vi "EPhysWork-Huet Model.vi"(3 "output control":T1, 4 "data":variant, 5 "X":dbl[](array[numeric]), 6 "a":dbl[](array[numeric])) -> (0 "error out":errorcluster, 1 "f'(X,a)":dbl[][](array[numeric]), 2 "f(X,a)":dbl[](array[numeric]))   [LabVIEW 2015]
doc: "Sum of three Gaussians, plus DC offset."
uses:
  <vilib>/gmath/NumericalOptimization/LM_output select.ctl
  <vilib>/gmath/NI_Gmath.lvlib
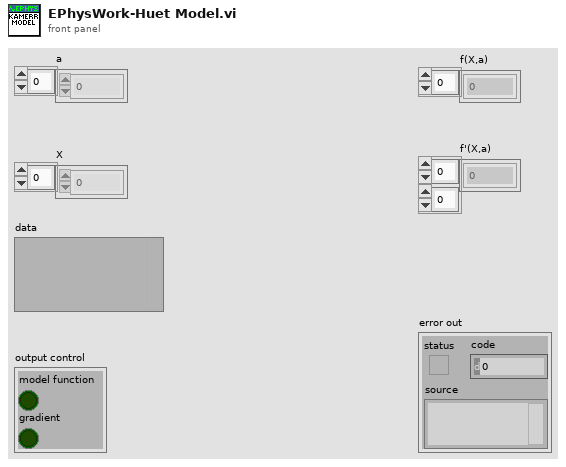
[diagram p1: front panel]
types:
  T1 = typedef "NI_Gmath.lvlib/LM_output select.ctl" = cluster{"model function":bool, "gradient":bool}
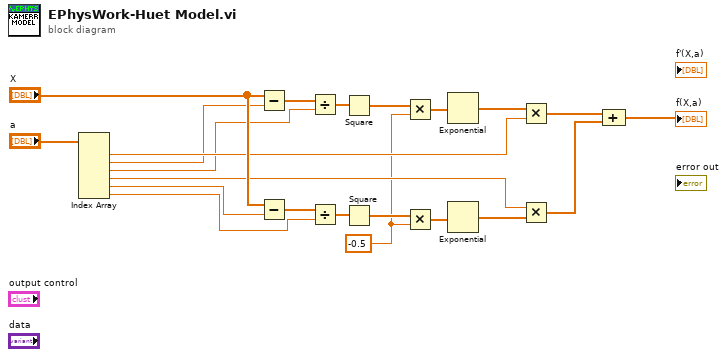
[diagram p0: block diagram]
diagram:
  w1 = -0.5
  n1 = Index Array(array="a") -> (element #1=w21:dbl, element #2=w20:dbl, element #3=w19:dbl, element #4=w18:dbl, element #5=w17:dbl, element #6=w16:dbl)  [unwired: 6 in]
  n2 = Subtract(x="X", y=w20) -> (x-y=w5:dbl[])
  n3 = Subtract(x="X", y=w17) -> (x-y=w4:dbl[])
  n4 = Divide(x=w5, y=w19) -> (x/y=w13:dbl[])
  n5 = Divide(x=w4, y=w16) -> (x/y=w10:dbl[])
  n6 = Square(x=w13) -> (x^2=w3:dbl[])
  n7 = Square(x=w10) -> (x^2=w2:dbl[])
  n8 = Multiply(x=w3, y=w1) -> (x*y=w7:dbl[])
  n9 = Multiply(x=w2, y=w1) -> (x*y=w6:dbl[])
  n10 = Exponential(1:w7) -> (0:w12:dbl[])
  n11 = Exponential(1:w6) -> (0:w11:dbl[])
  n12 = Multiply(x=w12, y=w21) -> (x*y=w9:dbl[])
  n13 = Multiply(x=w18, y=w11) -> (x*y=w8:dbl[])
  n14 = Compound Arithmetic op=ADD(w9, w8) -> (→"f(X,a)":dbl[])
